vi "BlackWhiteIdentification.vi"(1 "whiteBOND":dbl, 2 "BlackBOND":dbl) -> (0 "BlackThenWhite":bool)   [LabVIEW 2013]
panel:
  out "isWhite":bool
  out "isBlack":bool
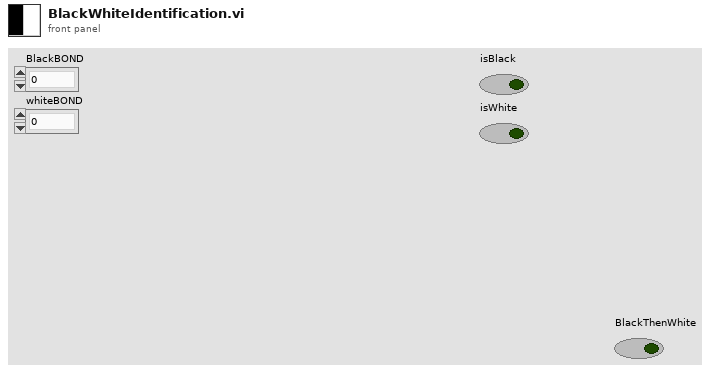
[diagram p1: front panel]
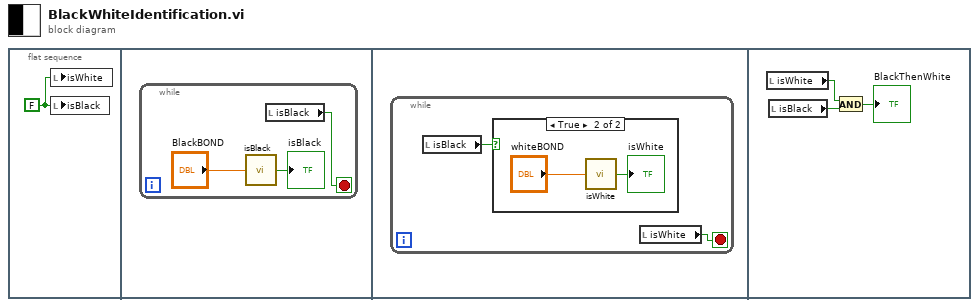
[diagram p0: block diagram]
diagram:
  n1 = flat-sequence {
    frame #0 {
      w1 = FALSE ("isWhite")
      n2 = local write "isWhite"(w1) -> ()
      n3 = local write "isBlack"(w1) -> ()
    }
    frame #1 {
      n4 = while {
        stop <- w2 stop-if-true
        n5 = call "isBlack.vi"("BlackBOND"="BlackBOND") -> ("isBlack"=→"isBlack":bool)
        n6 = local read "isBlack"() -> (w2:bool)
      }
    }
    frame #2 {
      n7 = while {
        stop <- w5 stop-if-true
        n8 = local read "isBlack"() -> (w6:bool)
        n9 = case shown="True" w6 {
          frame False {
          }
          frame True {
            n10 = call "isWhite.vi"("whiteBOND"="whiteBOND") -> ("isWhite"=→"isWhite":bool)
          }
        }
        n11 = local read "isWhite"() -> (w5:bool)
      }
    }
    frame #3 {
      n12 = local read "isWhite"() -> (w11:bool)
      n13 = local read "isBlack"() -> (w10:bool)
      n14 = And(x=w11, y=w10) -> (x .and. y?=→"BlackThenWhite":bool)
    }
  }
